vi "3_5_5.vi"() -> ()   [LabVIEW 2012]
panel:
  in  "Array":cluster{i32, i32}[](array[cluster])
  out "Array 3":cluster{i32, i32}[](array[cluster])
  in  "Numeric":i32
  in  "Array 2":i32[][](array[numeric])
  in  "stop":bool
  in  "OK Button":bool
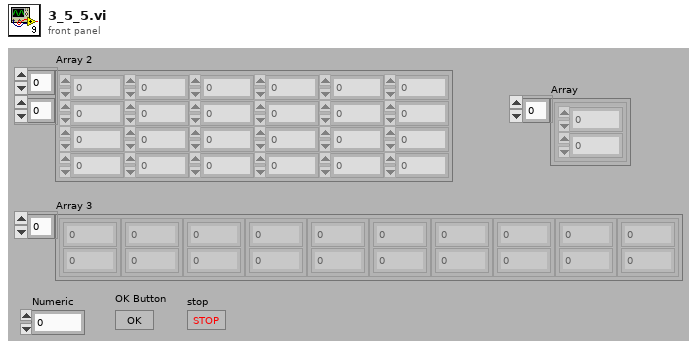
[diagram p1: front panel]
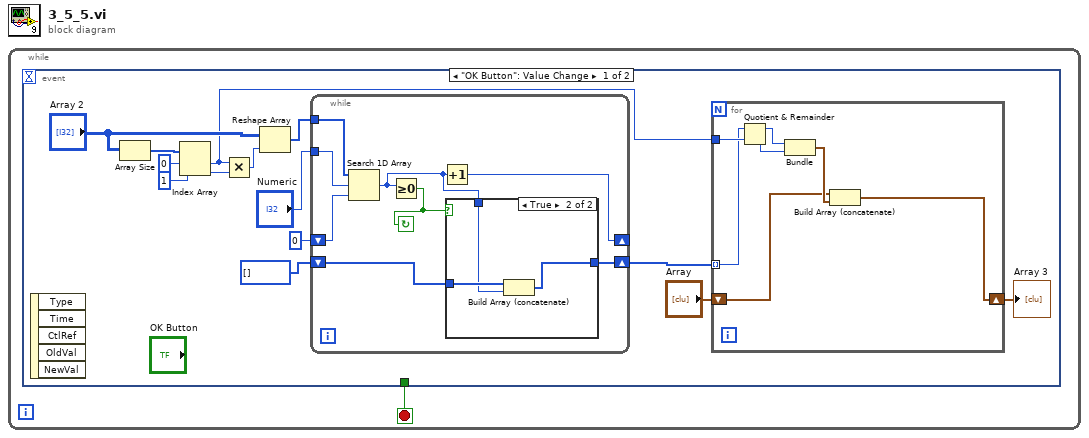
[diagram p0: block diagram]
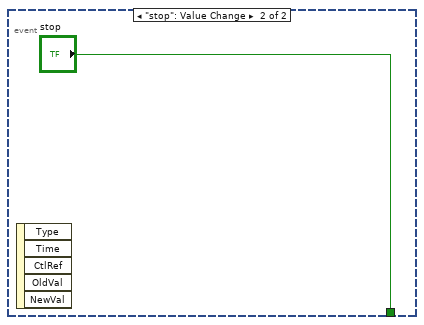
[diagram p3: hidden frame]
diagram:
  n1 = while {
    stop <- w1 stop-if-true
    n2 = event shown="[0] \"OK Button\": Value Change" {
      selector: _ -> [_ _]
      dyn-events: _ -> [_ _]
      timeout: _ -> [_ _]
      tunnel: [_ "stop"] -> w1
      event "OK Button": Value Change {
        n3 = event-data() -> ()  [unwired: 1 in, 5 out]
        n4 = Array Size(array="Array 2") -> (size(s)=w15:i32[])
        n5 = Index Array(array=w15, index #1=0 ("index"), index #2=1 ("index")) -> (element #1=w5:i32, element #2=w12:i32)
        n6 = Multiply(x=w5, y=w12) -> (x*y=w10:i32)
        n7 = Reshape Array("Array 2", w10) -> (w9:i32[])
        n8 = while {
          tunnel: w9 -> [w30]
          tunnel: "Numeric" -> [w29]
          shift-right: [w23] -> w4
          shift-left: i32[] [] -> [w25]
          shift-right: [w28] -> _
          shift-left: 0 -> [w27]
          stop <- w26 continue-if-true
          n9 = Search 1D Array(1D array=w30, element=w29, start index (0)=w27) -> (index of element=w24:i32)
          n10 = Greater Or Equal To 0?(x=w24) -> (x >= 0?=w26:bool)
          n11 = Increment(x=w24) -> (x+1=w28:i32)
          n12 = case shown="True" w26 {
            tunnel: w25 -> [w31 w34]
            tunnel: w24 -> [_ w33]
            tunnel: [w31 w32] -> w23
            frame False {
            }
            frame True {
              n13 = Build Array (concatenate)(w34, w33) -> (w32:i32[])
            }
          }
        }
        n14 = for {
          tunnel: w5 -> [w22]
          tunnel: w4 -> [w21] mode=indexing
          shift-right: [w16] -> w3
          shift-left: "Array" -> [w17]
          n15 = Quotient & Remainder(x=w21, y=w22) -> (x-y*floor(x/y)=w20:i32, floor(x/y)=w19:i32)
          n16 = Bundle(w20, w19) -> (w18:cluster{i32, i32})  [unwired: 1 in]
          n17 = Build Array (concatenate)(w17, w18) -> (w16:cluster{i32, i32}[])
        }
        "Array 3" <- w3
      }
      event "stop": Value Change {
        n18 = event-data() -> ()  [unwired: 1 in, 5 out]
      }
    }
  }
